vi "postodegrees.vi"(3 "Degrees @ Home (15.00)":dbl=15.0 format="%.2f", 4 "Ticks per degree (28571.43)":dbl=28571.43 format="%.2f", 5 "Ext Position":i32) -> (1 "Degrees":dbl=10.0 min=8.0 max=70.0 format="%.2f")   [LabVIEW 2015]
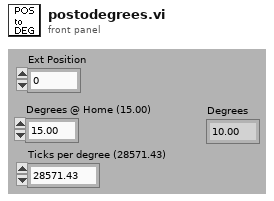
[diagram p1: front panel]
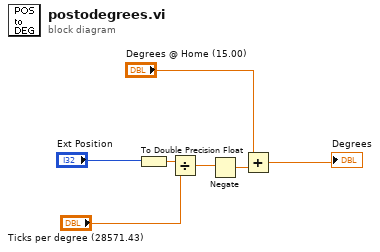
[diagram p0: block diagram]
diagram:
  n1 = To Double Precision Float(number="Ext Position") -> (double precision float=w7:dbl)
  n2 = Divide(x=w7, y="Ticks per degree (28571.43)") -> (x/y=w6:dbl)
  n3 = Negate(x=w6) -> (-x=w5:dbl)
  n4 = Add(x="Degrees @ Home (15.00)", y=w5) -> (x+y=→"Degrees":dbl)
